vi "Set Detection.vi"(8 "error in (no error)":errorcluster, 10 "Detection":T1=enum."Cy3 (LP550)", 11 "Virtual Microscope in":refnum<class "Virtual Microscope.lvclass">) -> (0 "error out":errorcluster, 3 "Virtual Microscope out":refnum<class "Virtual Microscope.lvclass">)   [LabVIEW 2015, in "Virtual Microscope.lvlib" / "Virtual Microscope.lvclass"]
uses:
  Virtual Microscope.lvclass
  Resources/Type Defs/Detection.ctl
  Virtual Microscope.lvclass/Virtual Microscope.ctl
  TE2000 Messages/Set Detection Msg/Set Detection Msg.lvclass/Set Detection Msg.ctl
  <vilib>/ActorFramework/Message Enqueuer/Message Enqueuer.lvclass/Message Enqueuer.ctl
  Eclipse TI Messages/Set Detection Msg/Set Detection Msg.lvclass/Set Detection Msg.ctl
  <vilib>/ActorFramework/Message Enqueuer/Enqueue.vi
  <vilib>/ActorFramework/Message Priority Queue/Priority Enqueue.vi
  TE2000 Messages/Set Detection Msg/Set Detection Msg.lvclass
  Eclipse TI Messages/Set Detection Msg/Set Detection Msg.lvclass
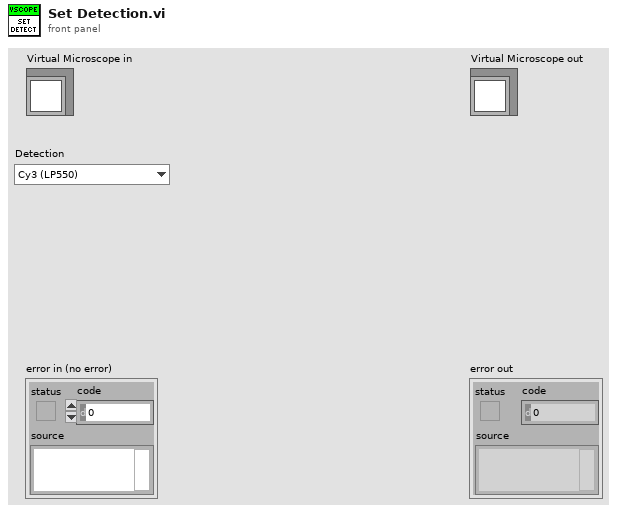
[diagram p1: front panel]
types:
  T1 = typedef "Detection.ctl" = enum16{"Cy2 (LP500)", "Cy3 (LP550)", "Cy5 (BP700/75)", "Cy3/Cy5 (BP590/40,700/60)", "No Filter", "Laser to Eyes"}
  T2 = typedef "Microscope Type.ctl" = enum16{"TE2000", "Eclipse Ti"}
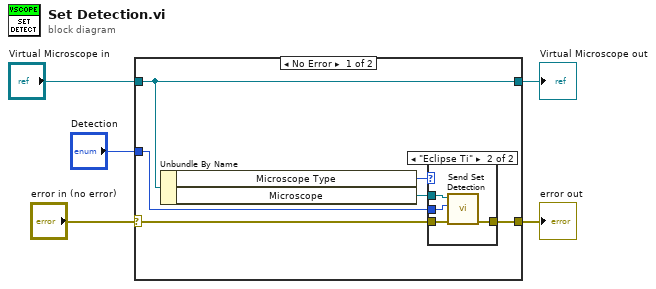
[diagram p0: block diagram]
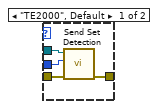
[diagram p2: hidden frame]
diagram:
  n1 = case shown="No Error" "error in (no error)" {
    selector: "error in (no error)" -> [w10 w21]
    tunnel: [w9 w21] -> w4
    tunnel: [w7 w20] -> w2
    tunnel: "Virtual Microscope in" -> [w7 w20]
    tunnel: "Detection" -> [w8 _]
    frame No Error {
      n2 = Unbundle By Name(w7) -> ("Microscope Type"=w11:T2, "Microscope"=w6:refnum<class "Message Enqueuer.lvclass">)
      n3 = case shown="\"Eclipse Ti\"" w11 {
        tunnel: w6 -> [w15 w19]
        tunnel: w10 -> [w14 w17]
        tunnel: [w13 w16] -> w9
        tunnel: w8 -> [w12 w18]
        frame "TE2000", Default {
          n4 = call "Send Set Detection.vi"("error in (no error)"=w14, "Detection"=w12, "Message Enqueuer"=w15) -> ("error out"=w13:errorcluster)  [unwired: 7 in, 1 out]
        }
        frame "Eclipse Ti" {
          n5 = call "Send Set Detection.vi"("error in (no error)"=w17, "Detection"=w18, "Message Enqueuer"=w19) -> ("error out"=w16:errorcluster)  [unwired: 7 in, 1 out]
        }
      }
    }
    frame Error {
    }
  }
  "error out" <- w4
  "Virtual Microscope out" <- w2
